vi "dfd_FXP Overflow.vi"   [LabVIEW 2017, in "NI_DigFilter_FXP.lvlib"]
uses:
  <vilib>/addons/Digital Filter Design/NI_DigFilter_FXP.lvlib
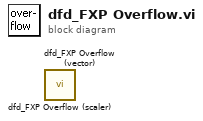
[diagram p0: block diagram]
diagram:
  n1 = call <vilib>:"dfd_FXP Overflow (scaler).vi"() -> ()  [unwired: 6 in, 3 out]
  n2 = call <vilib>:"dfd_FXP Overflow (vector).vi"() -> ()  [unwired: 6 in, 3 out]
